vi "Cache_Hierarchy Global.vi"() -> ()   [LabVIEW 2019, in "ClassLoader.lvlib"]
uses:
  ClassLoader.lvlib
panel:
  in  "Hierarchy":map{string, string[]}(c390)
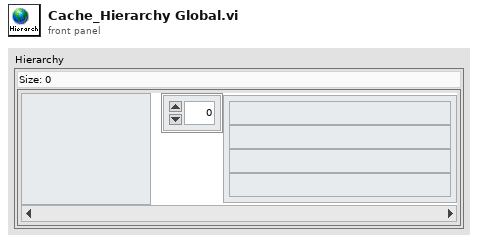
[diagram p1: front panel]
diagram:
